vi "Find Particle.vi"(7 "File Path":path, 8 "error in":errorcluster, 9 "Camera Image":T1, 10 "From File":bool, 11 "R/G/B":cluster{"Lower value":i32, "Upper value":i32}[](array[cluster])) -> (0 "error out":errorcluster, 1 "Particle Report":T2(array[cluster]) {"Orientation" format="%.2f"; "Dimensions"."Height" format="%.2f"; "Dimensions"."Width" format="%.2f"; "Center of Mass"."Y" format="%.2f"; "Center of Mass"."X" format="%.2f"; "Bounding Rect"."Bottom" format="%.2f"; "Bounding Rect"."Right" format="%.2f"; "Bounding Rect"."Top" format="%.2f"; "Bounding Rect"."Left" format="%.2f"; "Number of Holes" format="%.2f"; "Area" format="%.2f"}, 2 "Thresholded Image":T1(plugin-control), 3 "Base Image":T1(plugin-control), 5 "Number of Particles":i32)   [LabVIEW 2017]
uses:
  <vilib>/vision/Image Controls.llb/IMAQ Image.ctl
  <vilib>/vision/NI_Vision_Development_Module.lvlib
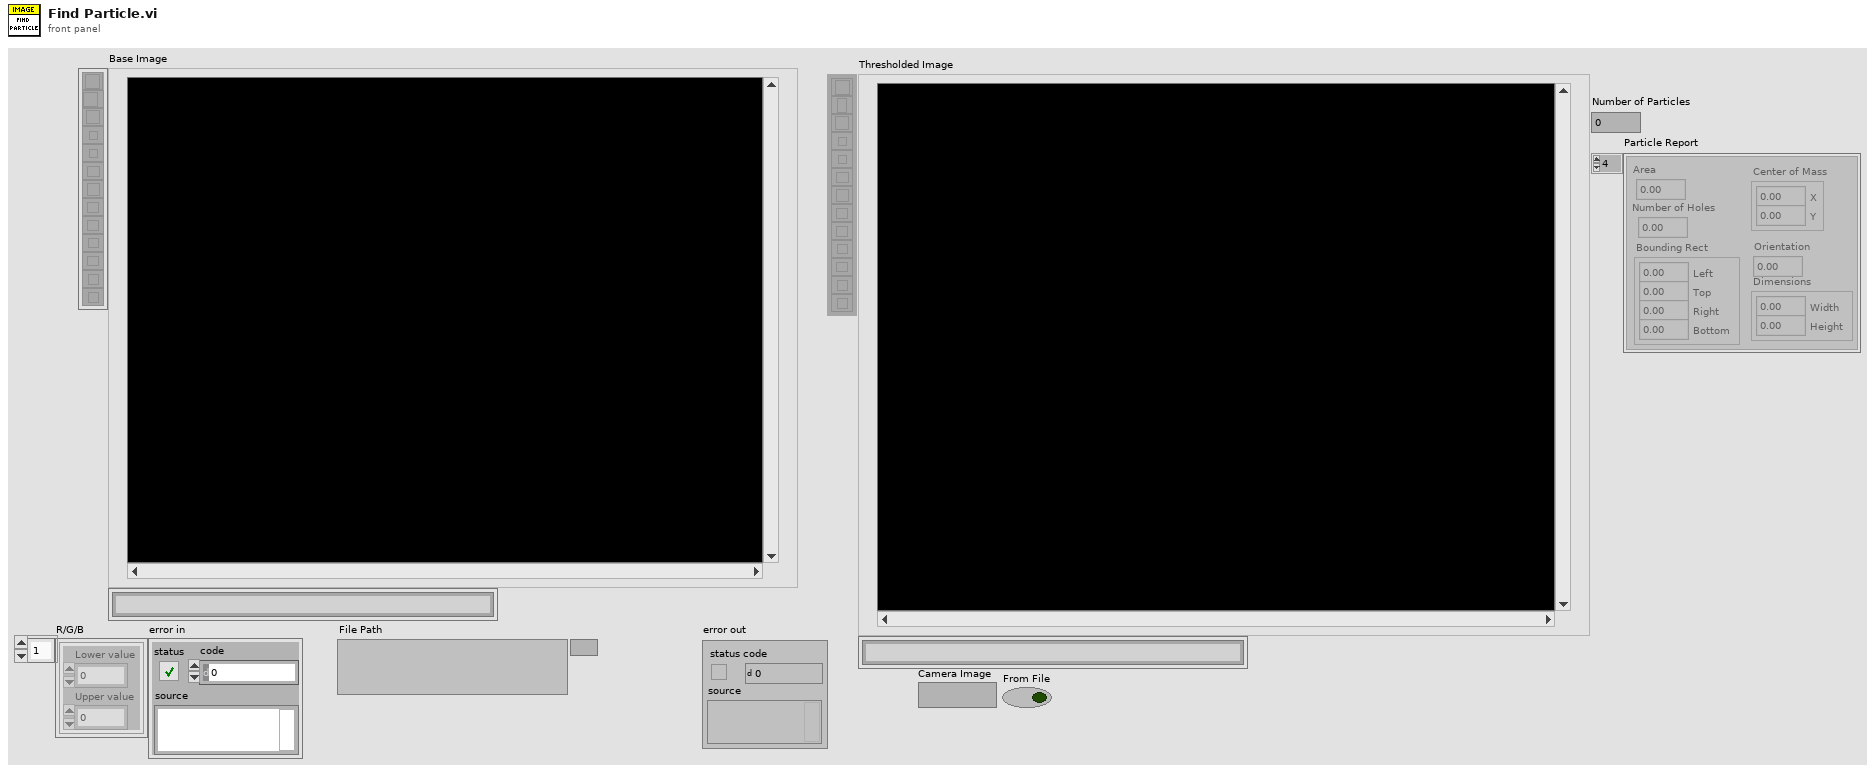
[diagram p1: front panel]
types:
  T1 = typedef "IMAQ Image.ctl" = refnum<image>
  T2 = cluster{"Area":dbl, "Number of Holes":dbl, "Bounding Rect":cluster{"Left":dbl, "Top":dbl, "Right":dbl, "Bottom":dbl}, "Center of Mass":cluster{"X":dbl, "Y":dbl}, "Orientation":dbl, "Dimensions":cluster{"Width":dbl, "Height":dbl}}[]
  T3 = typedef "Image Type" = u32
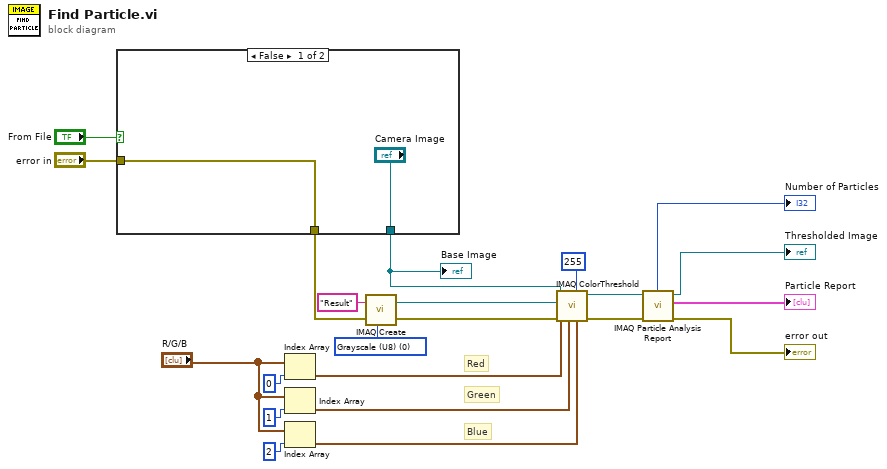
[diagram p0: block diagram]
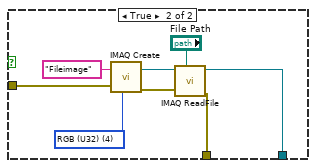
[diagram p2: hidden frame]
diagram:
  w21 = T3 0 items=["Grayscale (U8)", "Grayscale (I16)", "Grayscale (SGL)", "Complex (CSG)", "RGB (U32)", "HSL (U32)", "RGB (U64)", "Grayscale (U16)"] ("Image Type")
  # "Blue"
  # "Green"
  # "Red"
  n1 = case shown="False" "From File" {
    tunnel: ["Camera Image" w28] -> w8
    tunnel: [w23 w27] -> w3
    tunnel: "error in" -> [w23 w26]
    frame False {
    }
    frame True {
      w30 = T3 4 items=["Grayscale (U8)", "Grayscale (I16)", "Grayscale (SGL)", "Complex (CSG)", "RGB (U32)", "HSL (U32)", "RGB (U64)", "Grayscale (U16)"] ("Image Type")
      n2 = call "IMAQ Create"("Image Name"="Fileimage", "Image Type"=w30, "error in (no error)"=w26) -> ("New Image"=w32:T1, "error out"=w31:errorcluster)  [unwired: 2 in]
      n3 = call "IMAQ ReadFile"("File Path"="File Path", "error in (no error)"=w31, "Image"=w32) -> ("error out"=w27:errorcluster, "Image Out"=w28:T1)  [unwired: 4 in, 3 out]
    }
  }
  "Base Image" <- w8
  n4 = Index Array(array="R/G/B", index=0) -> (element=w11:cluster{"Lower value":i32, "Upper value":i32})
  n5 = Index Array(array="R/G/B", index=1) -> (element=w10:cluster{"Lower value":i32, "Upper value":i32})
  n6 = Index Array(array="R/G/B", index=2) -> (element=w9:cluster{"Lower value":i32, "Upper value":i32})
  n7 = call "IMAQ Create"("Image Name"="Result", "Image Type"=w21, "error in (no error)"=w3) -> ("New Image"=w20:T1, "error out"=w5:errorcluster)  [unwired: 2 in]
  n8 = call "IMAQ ColorThreshold"("Blue or Luma or Val or Inten Range"=w9, "Replace Value"=255, "Green or Sat Range"=w10, "error in (no error)"=w5, "Red or Hue Range"=w11, "Image Dst"=w20, "Image Src"=w8) -> ("error out"=w4:errorcluster, "Image Dst Out"=w18:T1)  [unwired: 3 in]
  n9 = call "IMAQ Particle Analysis Report"("error in (no error)"=w4, "Image"=w18) -> ("error out"=→"error out":errorcluster, "Particle Reports (Pixels)"=→"Particle Report":T2, "Image Out (duplicate)"=→"Thresholded Image":T1, "Number of Particles"=→"Number of Particles":i32)  [unwired: 4 in, 2 out]
